vi "Freefield-Restore Defaults.vi"() -> (8 "Parameters":T1)   [LabVIEW 2020]
uses:
  Typedefs/FF-Parameters.ctl
  Common VIs/Typedefs/CAL-Stimulus.ctl
  Common VIs/Typedefs/CAL-Response.ctl
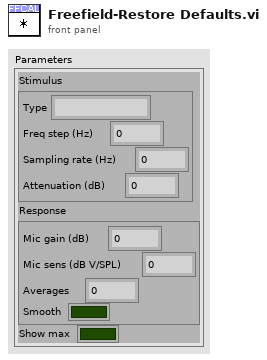
[diagram p1: front panel]
types:
  T1 = typedef "FF-Parameters.ctl" = cluster{"Stimulus":T2, "Response":T3, "Show max":bool}
  T2 = typedef "CAL-Stimulus.ctl" = cluster{"Type":string, "Freq step (Hz)":dbl, "Sampling rate (Hz)":dbl, "Attenuation (dB)":dbl}
  T3 = typedef "CAL-Response.ctl" = cluster{"Mic gain (dB)":dbl, "Mic sens (dB V/SPL)":dbl, "Averages":i32, "Smooth":bool}
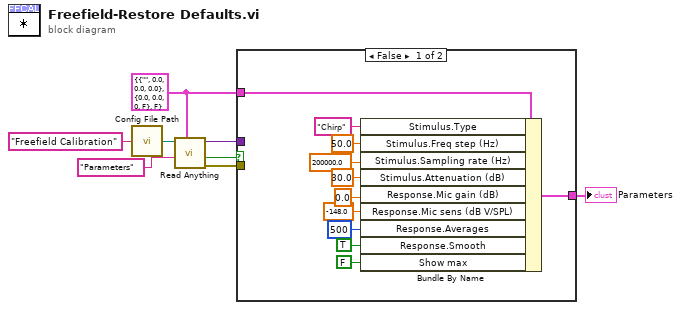
[diagram p0: block diagram]
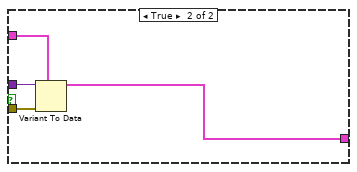
[diagram p2: hidden frame]
diagram:
  w3 = T1 {"Stimulus"={"Type"="", "Freq step (Hz)"=0.0, "Sampling rate (Hz)"=0.0, "Attenuation (dB)"=0.0}, "Response"={"Mic gain (dB)"=0.0, "Mic sens (dB V/SPL)"=0.0, "Averages"=0, "Smooth"=FALSE}, "Show max"=FALSE} ("Parameters")
  n1 = call "Config File Path.vi"("AppName"="Freefield Calibration") -> ("Default config file name"=w8:path)
  n2 = call "Read Anything.vi"("Type of Anything"=w3, "Section Name (Name of \"Type of Anything\")"="Parameters" ("Section Name (Name of \"Type of Anything\")"), "Path (dialog)"=w8) -> ("Error Out"=w6:errorcluster, "Found?"=w5:bool, "Anything"=w4:variant)  [unwired: 6 in]
  n3 = case shown="False" w5 {
    tunnel: w6 -> [_ w23]
    tunnel: w4 -> [_ w22]
    tunnel: w3 -> [w19 w21]
    tunnel: [w18 w20] -> w2
    frame False {
      n4 = Bundle By Name(cluster=w19, "Stimulus.Type"="Chirp", "Stimulus.Freq step (Hz)"=50.0, "Stimulus.Sampling rate (Hz)"=200000.0, "Stimulus.Attenuation (dB)"=30.0, "Response.Mic gain (dB)"=0.0, "Response.Mic sens (dB V/SPL)"=-148.0, "Response.Averages"=500, "Response.Smooth"=TRUE, "Show max"=FALSE ("Response.Show max")) -> (w18:T1)
    }
    frame True {
      n5 = Variant To Data(error in=w23, type=w21, Variant=w22) -> (data=w20:T1)  [unwired: 1 out]
    }
  }
  "Parameters" <- w2
